vi "GetMetaData.vi"(8 "error in (no error)":errorcluster, 11 "VISA Input":refnum<visa-resource-name>) -> (0 "error out":errorcluster, 1 "Metadata 3":string, 2 "Metadata 2":string, 3 "VISA Output":refnum<visa-resource-name>, 4 "Error?":bool, 5 "Metadata 1":string)   [LabVIEW 2015]
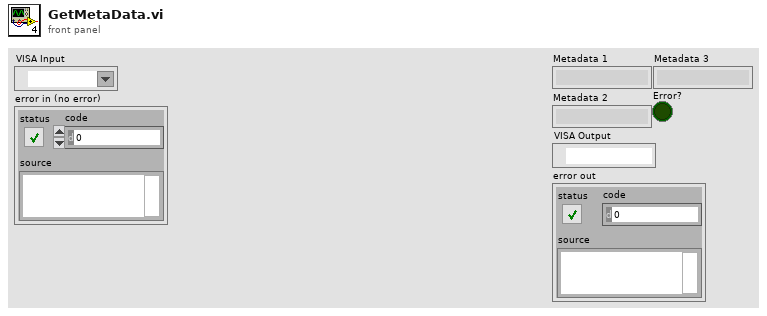
[diagram p1: front panel]
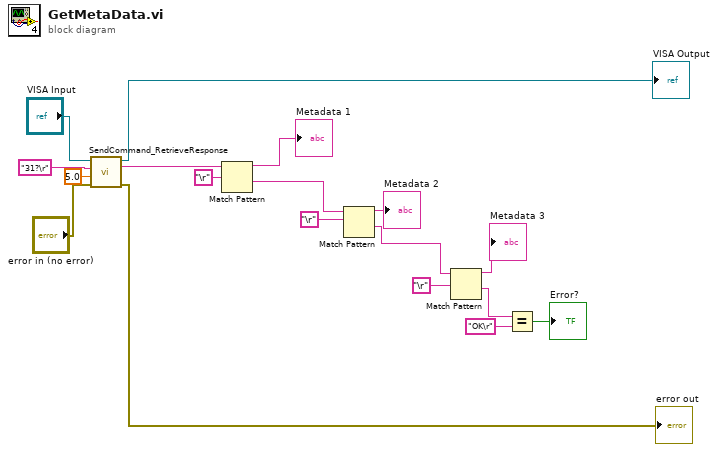
[diagram p0: block diagram]
diagram:
  n1 = call "SendCommand_RetrieveResponse.vi"("error in (no error)"="error in (no error)", "Timeout (Seconds)"=5.0, "Input Command"="31?\r", "VISA Input"="VISA Input") -> ("error out"=→"error out":errorcluster, "System Response"=w14:string, "VISA Output"=→"VISA Output":refnum<visa-resource-name>)  [unwired: 4 in, 1 out]
  n2 = Match Pattern(string=w14, regular expression="\r") -> (before substring=→"Metadata 1":string, after substring=w8:string)  [unwired: 1 in, 2 out]
  n3 = Match Pattern(string=w8, regular expression="\r") -> (before substring=→"Metadata 2":string, after substring=w9:string)  [unwired: 1 in, 2 out]
  n4 = Match Pattern(string=w9, regular expression="\r") -> (before substring=→"Metadata 3":string, after substring=w5:string)  [unwired: 1 in, 2 out]
  n5 = Equal?(x=w5, y="OK\r") -> (x = y?=→"Error?":bool)
